vi "Main VI.vi"() -> ()   [LabVIEW 2017]
uses:
  State Machine Controler.ctl
  <vilib>/DAQmx/read.llb/DAQmx Read (Analog 1D DBL 1Chan NSamp).vi
  <vilib>/DAQmx/write.llb/DAQmx Write (Digital 1D Bool NChan 1Samp 1Line).vi
  <vilib>/DAQmx/miscellaneous.llb/DAQmx Fill In Error Info.vi
  <vilib>/DAQmx/create/channels.llb/DAQmx Create Channel (DO-Digital Output).vi
  <vilib>/DAQmx/configure/timing.llb/DAQmx Timing (Sample Clock).vi
panel:
  in  "BSL Flash 2":bool
  out "Auto Command indicator 3":u32
  out "Waveform Graph":dbl[](graph)
  out "output cluster":cluster{"x/y 2":dbl}(graph)
  out "Current loop count":i32
  out "Current value":dbl
  in  "physical channels":tag
  in  "error in":errorcluster
  out "Auto Command indicator 2":u32
  in  "BSL Flash wait time":u32=75
  out "Manual down  ON time":u32
  out "Auto Command indicator":u32
  out "Numeric":i32
  out "Auot Travel Time Indicator":u32
  in  "Auto Travel Time Controler":u32
  in  "Manual Up":bool
  in  "Manual Down":bool
  in  "Clamp/ Unclamp":bool
  out "State":T1
  in  "Auto Down Command":u32=75
  in  "Manual UP":bool
  in  "Stop":bool
  in  "BSL Flash":bool
  in  "Auto Down":bool
  in  "Auto UP":bool
  in  "Manual DOWN":bool
  # "Std Motor"
  # "Anti-Pinch Motor"
  # "min 87"
  # "max=526"
  # "max 537"
  # "Min=75"
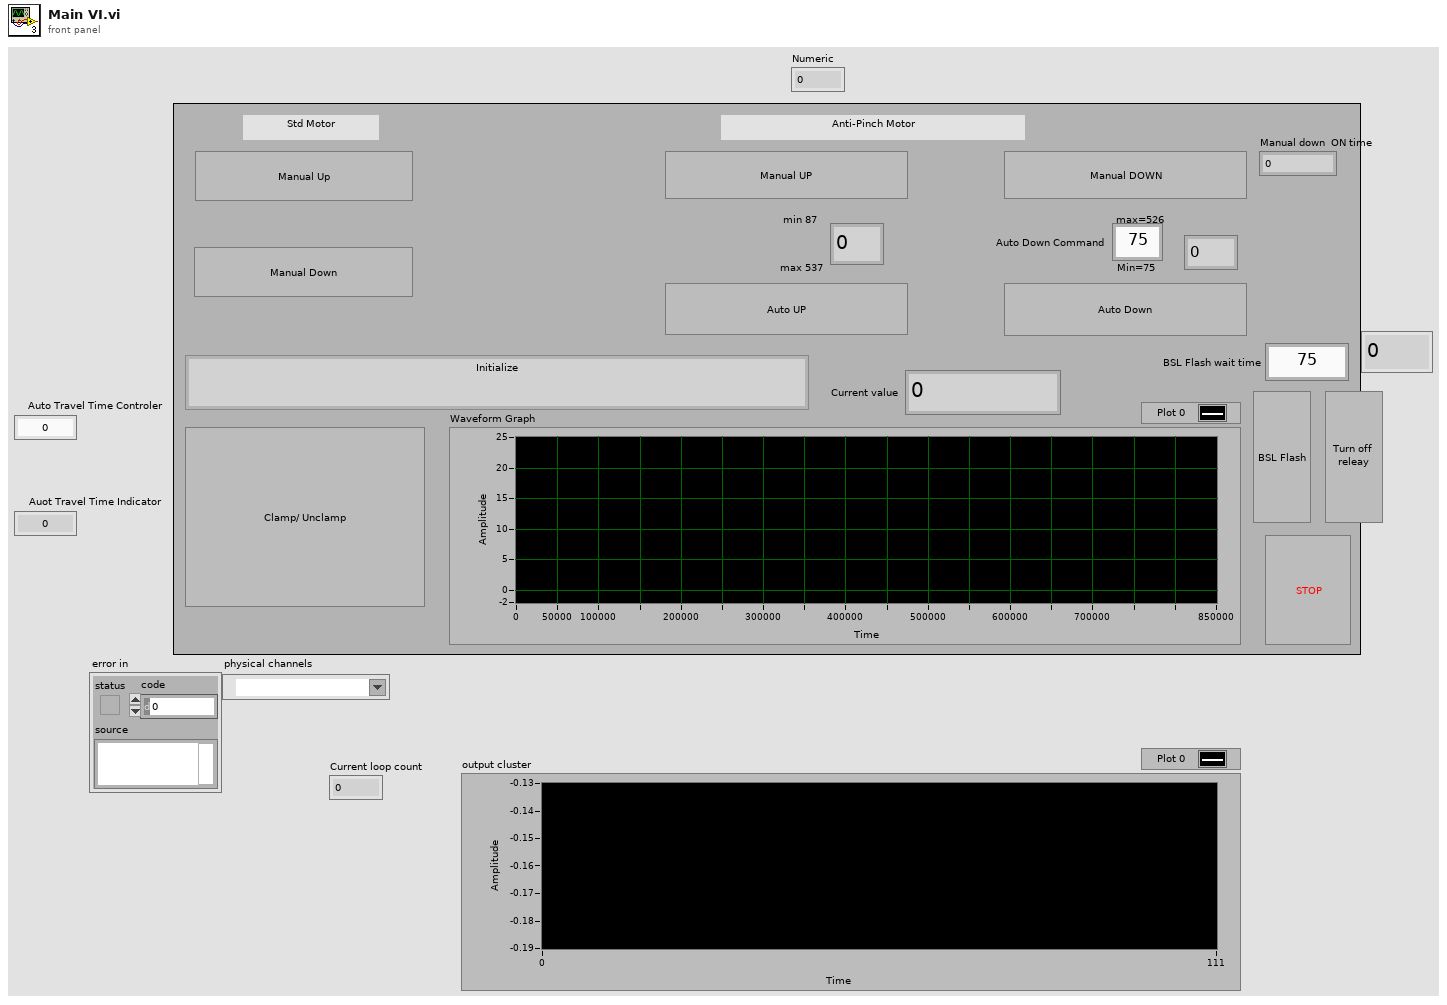
[diagram p1: front panel]
types:
  T1 = typedef "State Machine Controler.ctl" = enum16{"Initialize", "Wait for Action", "Manual Up AP", "Manual Up Std", "Manual Stop", "Manual Down AP", "Manual Down Std", "Auto Up", "Auto Down", "Auto Mode Down", "Auto Mode Up", "Auto Mode Waiting", "BSL Flash", "Stop"}
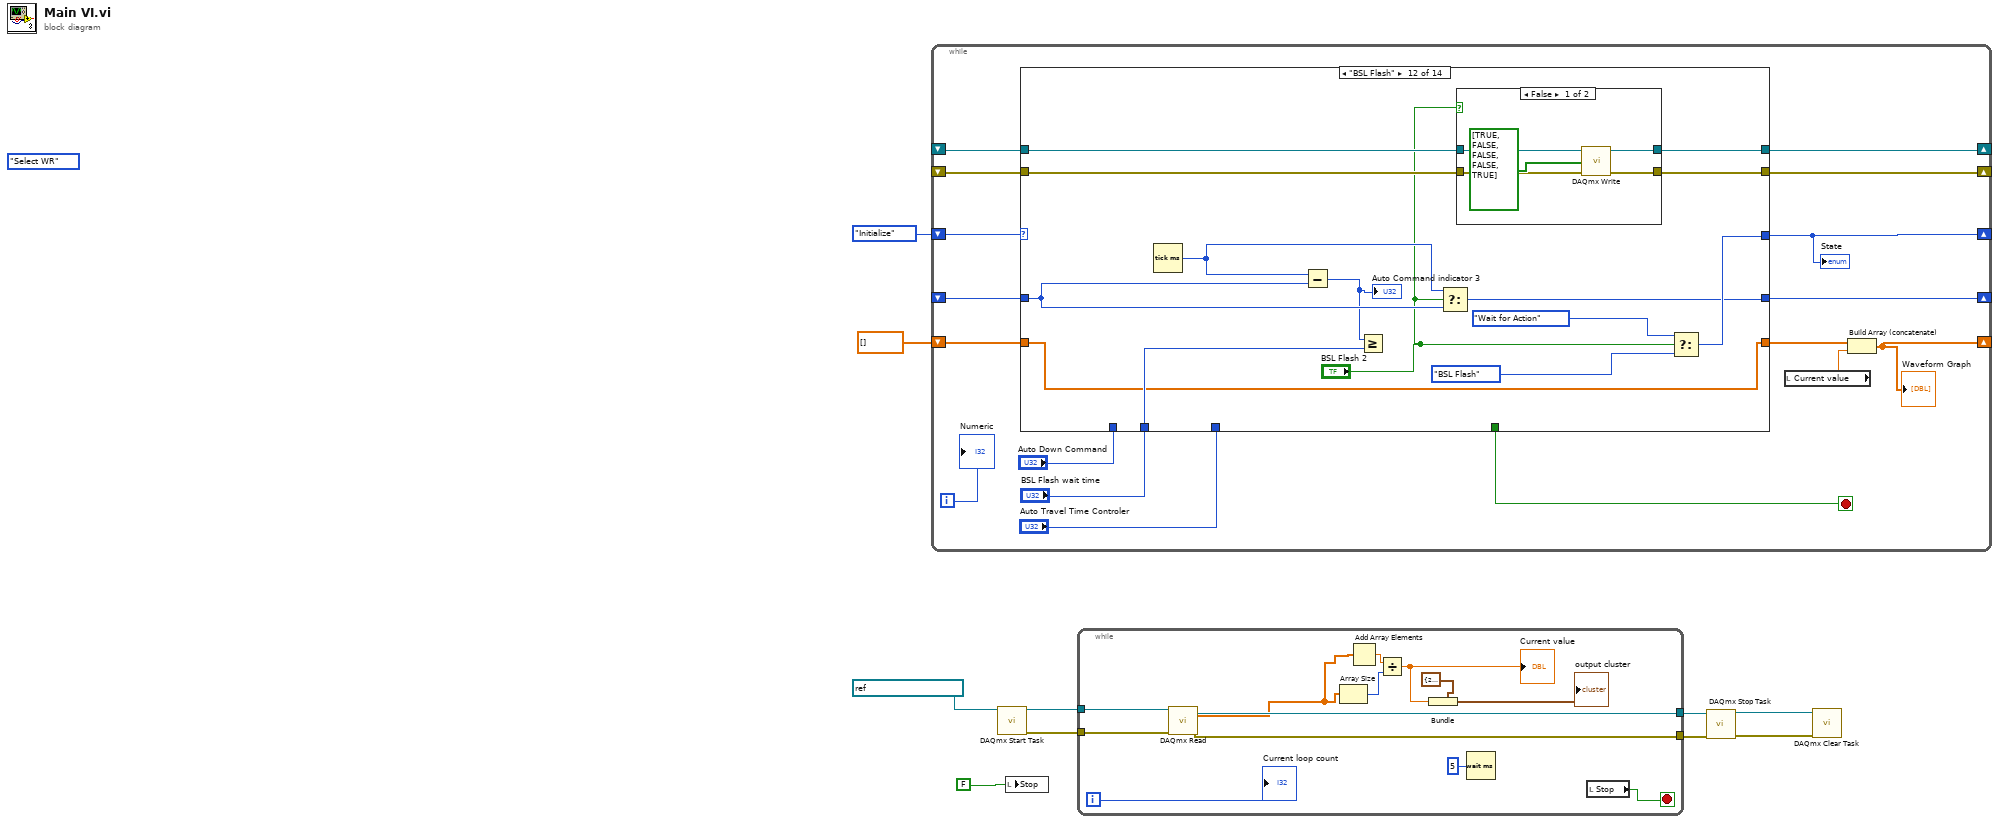
[diagram p0: block diagram]
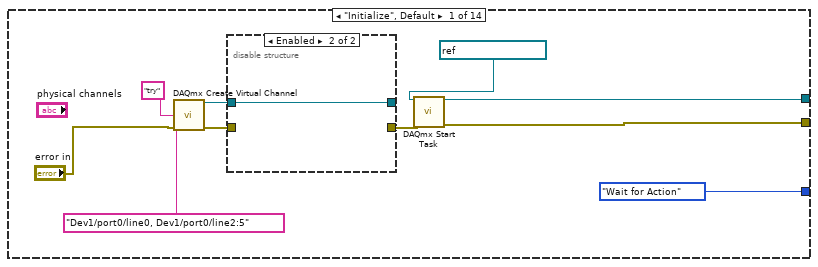
[diagram p2: hidden frame]
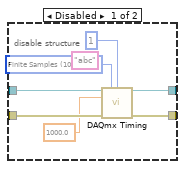
[diagram p3: hidden frame]
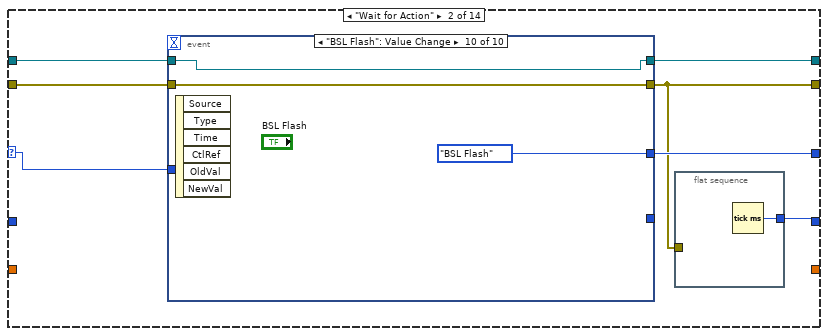
[diagram p4: hidden frame]
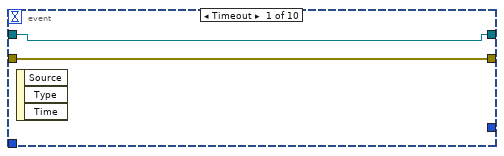
[diagram p5: hidden frame]
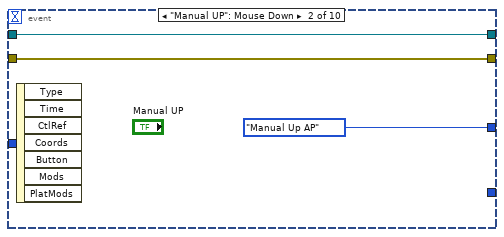
[diagram p6: hidden frame]
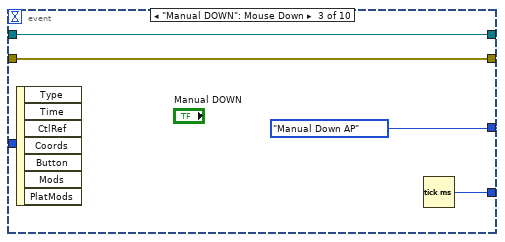
[diagram p7: hidden frame]
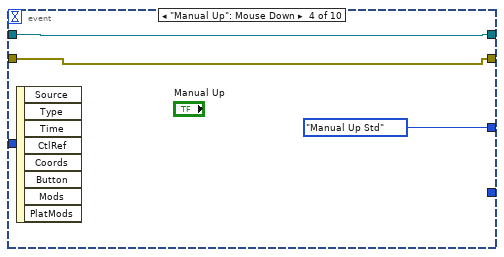
[diagram p8: hidden frame]
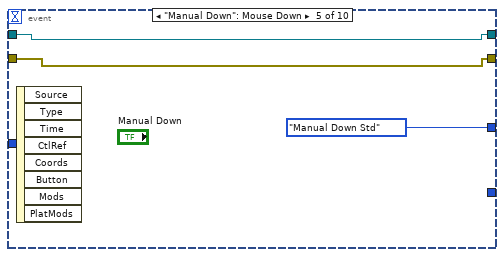
[diagram p9: hidden frame]
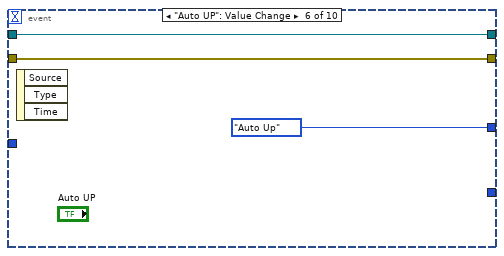
[diagram p10: hidden frame]
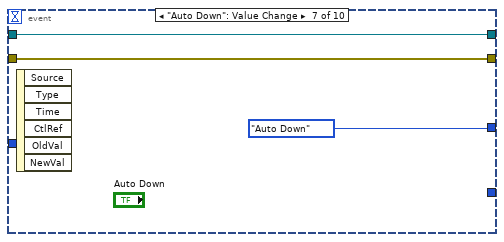
[diagram p11: hidden frame]
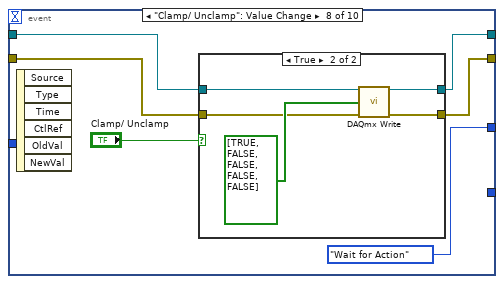
[diagram p12: hidden frame]
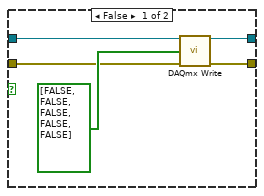
[diagram p13: hidden frame]
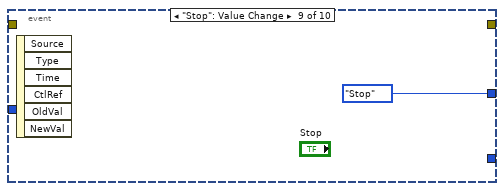
[diagram p14: hidden frame]
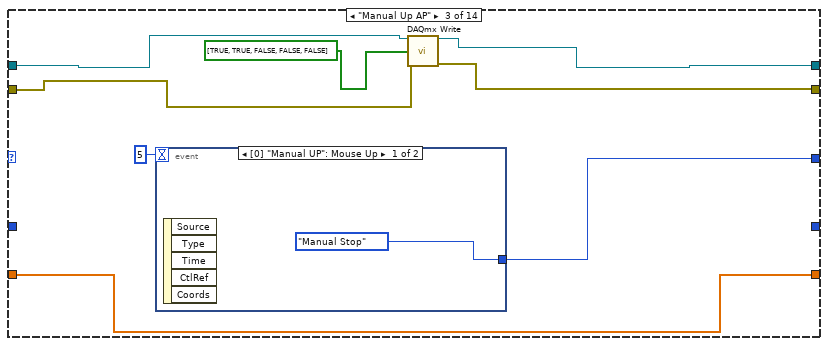
[diagram p15: hidden frame]
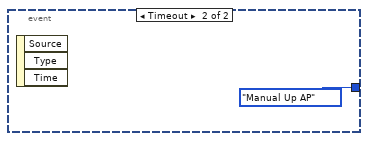
[diagram p16: hidden frame]
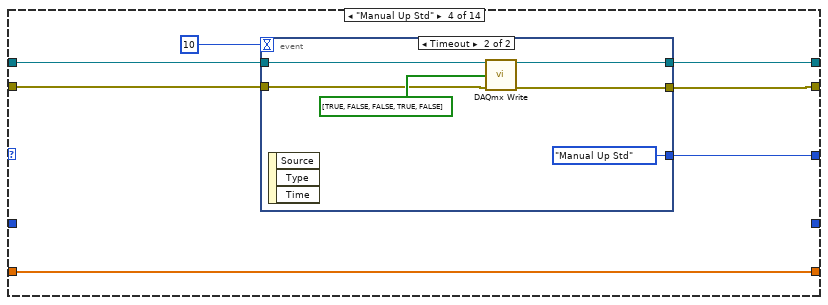
[diagram p17: hidden frame]
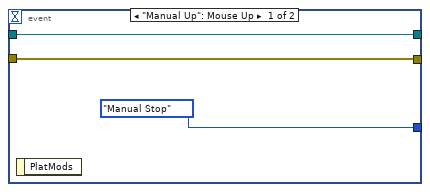
[diagram p18: hidden frame]
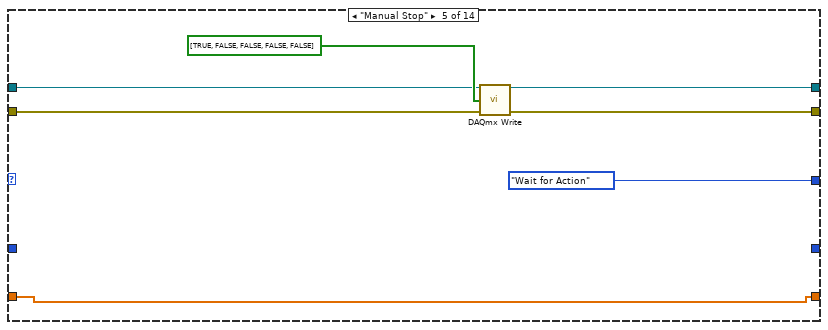
[diagram p19: hidden frame]
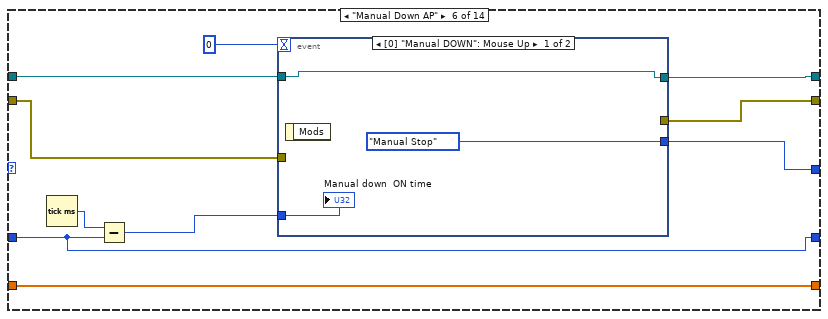
[diagram p20: hidden frame]
diagram:
  (unwired) enum16{"Select WR"}."Select WR"
  n1 = while {
    shift-right: [w18] -> _
    shift-left: State_Machine_Controler."Initialize" -> [w27]
    shift-right: [w22] -> _
    shift-left: _ -> [w24]
    shift-right: [w21] -> _
    shift-left: _ -> [w23]
    shift-right: [w26] -> _
    shift-left: _ -> [w25]
    shift-right: [w11] -> _
    shift-left: dbl[] [] -> [w14]
    i -> [w16]
    stop <- w20 stop-if-true
    n2 = case shown="\"BSL Flash\"" w27 {
      selector: w27 -> [_ w49 _ _ _ _ _ _ _ _ _ _ _ _]
      tunnel: [State_Machine_Controler."Wait for Action" w52 w102 w111 State_Machine_Controler."Wait for Action" w137 w153 State_Machine_Controler."Auto Mode Up" State_Machine_Controler."Auto Mode Down" w191 w212 w233 w252 State_Machine_Controler."Stop"] -> w18
      tunnel: w24 -> [_ w51 w100 w110 w126 w136 w152 w168 w178 w188 w210 w231 w258 w275]
      tunnel: w23 -> [_ w50 w99 w108 w125 w134 w150 w165 w177 w187 w209 w230 w257 w274]
      tunnel: [_ w46 _ _ _ w129 _ w170 w173 w182 w204 w226 w245 _] -> w26
      tunnel: w25 -> [_ _ _ _ _ w129 _ _ _ w181 w203 w225 w245 _]
      tunnel: "Auto Down Command" -> [_ _ _ _ _ _ _ _ _ w190 _ _ _ _]
      tunnel: [w36 w48 w97 w109 w123 w135 w151 w167 w175 w186 w208 w229 w255 _] -> w22
      tunnel: [w37 w47 w98 w107 w124 w133 w149 w164 w176 w185 w207 w228 w256 w271] -> w21
      tunnel: [_ _ _ _ _ _ _ _ _ _ _ _ _ TRUE ("Stop")] -> w20
      tunnel: "Auto Travel Time Controler" -> [_ _ _ _ _ _ _ _ _ _ _ _ w259 _]
      tunnel: "BSL Flash wait time" -> [_ _ _ _ _ _ _ _ _ _ w202 w224 _ _]
      tunnel: w14 -> [_ _ w96 w105 w121 w128 w147 w163 w171 w179 w200 w222 w251 _]
      tunnel: [_ _ w96 w105 w121 w128 w147 w163 w171 w179 w200 w222 w251 _] -> w12
      frame "Initialize", Default {
        n3 = call-poly <vilib>:"DAQmx Create Virtual Channel.vi"("lines"=tag "Dev1/port0/line0, Dev1/port0/line2:5", "name to assign"="try", "error in"="error in") -> ("task out"=w31:refnum<k21>, "error out"=w30:errorcluster)  [unwired: 11 in]
        n4 = disable-structure shown="Enabled" {
          disable-tunnel: w31 -> [w44 w45]
          disable-tunnel: [w43 w45] -> _
          disable-tunnel: w30 -> [w41 _]
          disable-tunnel: [w40 _] -> w29
          frame Disabled {
            w42 = 10178 items=["Finite Samples"=10178, "Continuous Samples"=10123, "Hardware Timed Single Point"=12522] ("sample mode")
            (unwired) "abc" ("new task name")
            n5 = call-poly <vilib>:"DAQmx Timing.vi"("task/channels in"=w44, "sample mode"=w42, "samples per channel"=1, "rate"=1000.0, "error in"=w41) -> ("task out"=w43:refnum<k21>, "error out"=w40:errorcluster)  [unwired: 9 in]
          }
          frame Enabled {
          }
        }
        n6 = call <vilib>:"DAQmx Start Task.vi"("task/channels in"=refnum<k21> "Test AP UP_DN", "error in"=w29) -> ("task out"=w36:refnum<k21>, "error out"=w37:errorcluster)  [unwired: 12 in]
      }
      frame "Wait for Action" {
        n7 = event shown="[9] \"BSL Flash\": Value Change" {
          selector: _ -> [_ _ _ _ _ _ _ _ _ _]
          dyn-events: _ -> [_ _ _ _ _ _ _ _ _ _]
          timeout: _ -> [_ _ _ _ _ _ _ _ _ _]
          tunnel: [_ State_Machine_Controler."Manual Up AP" State_Machine_Controler."Manual Down AP" State_Machine_Controler."Manual Up Std" State_Machine_Controler."Manual Down Std" State_Machine_Controler."Auto Up" State_Machine_Controler."Auto Down" State_Machine_Controler."Wait for Action" State_Machine_Controler."Stop" State_Machine_Controler."BSL Flash"] -> w52
          tunnel: w51 -> [w55 w57 w61 w64 w67 w69 w74 w80 _ w93]
          tunnel: w50 -> [w54 w56 w60 w63 w66 w70 w73 w78 _ w92]
          tunnel: [w55 w57 w61 w64 w67 w69 w74 w79 _ w93] -> w48
          tunnel: [w54 w56 w60 w63 w66 w70 w73 w77 _ w92] -> w47
          tunnel: w49 -> [_ _ _ _ _ _ _ _ _ _]
          tunnel: [_ _ w59 _ _ _ _ _ _ _] -> _
          event Timeout {
            n8 = event-data() -> ()  [unwired: 1 in, 3 out]
          }
          event "Manual UP": Mouse Down {
            n9 = event-data() -> ()  [unwired: 1 in, 7 out]
          }
          event "Manual DOWN": Mouse Down {
            n10 = event-data() -> ()  [unwired: 1 in, 7 out]
            n11 = Tick Count (ms)() -> (millisecond timer value=w59:u32)
          }
          event "Manual Up": Mouse Down {
            n12 = event-data() -> ()  [unwired: 1 in, 8 out]
          }
          event "Manual Down": Mouse Down {
            n13 = event-data() -> ()  [unwired: 1 in, 8 out]
          }
          event "Auto UP": Value Change {
            n14 = event-data() -> ()  [unwired: 1 in, 3 out]
          }
          event "Auto Down": Value Change {
            n15 = event-data() -> ()  [unwired: 1 in, 6 out]
          }
          event "Clamp/ Unclamp": Value Change {
            n16 = event-data() -> ()  [unwired: 1 in, 6 out]
            n17 = case shown="True" "Clamp/ Unclamp" {
              tunnel: w80 -> [w84 w89]
              tunnel: [w83 w88] -> w79
              tunnel: w78 -> [w82 w87]
              tunnel: [w81 w86] -> w77
              frame False {
                n18 = call-poly <vilib>:"DAQmx Write.vi"("task/channels in"=w84, "data"=bool[] [FALSE, FALSE, FALSE, FALSE, FALSE], "error in"=w82) -> ("task out"=w83:refnum<k21>, "error out"=w81:errorcluster)  [unwired: 10 in, 1 out]
              }
              frame True {
                n19 = call-poly <vilib>:"DAQmx Write.vi"("task/channels in"=w89, "data"=bool[] [TRUE, FALSE, FALSE, FALSE, FALSE], "error in"=w87) -> ("task out"=w88:refnum<k21>, "error out"=w86:errorcluster)  [unwired: 10 in, 1 out]
              }
            }
          }
          event "Stop": Value Change {
            n20 = event-data() -> ()  [unwired: 1 in, 6 out]
          }
          event "BSL Flash": Value Change {
            n21 = event-data() -> ()  [unwired: 1 in, 6 out]
          }
        }
        n22 = flat-sequence {
          tunnel: w47 -> [_]
          tunnel: [w53] -> w46
          frame #0 {
            n23 = Tick Count (ms)() -> (millisecond timer value=w53:u32)
          }
        }
      }
      frame "Manual Up AP" {
        n24 = event shown="[0] \"Manual UP\": Mouse Up" {
          selector: _ -> [_ _]
          dyn-events: _ -> [_ _]
          timeout: 5 -> [_ _]
          tunnel: [State_Machine_Controler."Manual Stop" State_Machine_Controler."Manual Up AP"] -> w102
          event "Manual UP": Mouse Up {
            n25 = event-data() -> ()  [unwired: 1 in, 5 out]
          }
          event Timeout {
            n26 = event-data() -> ()  [unwired: 1 in, 3 out]
          }
        }
        n27 = call-poly <vilib>:"DAQmx Write.vi"("task/channels in"=w100, "data"=bool[] [TRUE, TRUE, FALSE, FALSE, FALSE], "error in"=w99) -> ("task out"=w97:refnum<k21>, "error out"=w98:errorcluster)  [unwired: 10 in, 1 out]
      }
      frame "Manual Up Std" {
        n28 = event shown="[1] Timeout" {
          selector: _ -> [_ _]
          dyn-events: _ -> [_ _]
          timeout: 10 -> [_ _]
          tunnel: [State_Machine_Controler."Manual Stop" State_Machine_Controler."Manual Up Std"] -> w111
          tunnel: w110 -> [w113 w119]
          tunnel: [w113 w118] -> w109
          tunnel: w108 -> [w112 w117]
          tunnel: [w112 w116] -> w107
          event "Manual Up": Mouse Up {
            n29 = event-data() -> ()  [unwired: 1 in, 1 out]
          }
          event Timeout {
            n30 = event-data() -> ()  [unwired: 1 in, 3 out]
            n31 = call-poly <vilib>:"DAQmx Write.vi"("task/channels in"=w119, "data"=bool[] [TRUE, FALSE, FALSE, TRUE, FALSE], "error in"=w117) -> ("task out"=w118:refnum<k21>, "error out"=w116:errorcluster)  [unwired: 10 in, 1 out]
          }
        }
      }
      frame "Manual Stop" {
        n32 = call-poly <vilib>:"DAQmx Write.vi"("task/channels in"=w126, "data"=bool[] [TRUE, FALSE, FALSE, FALSE, FALSE], "error in"=w125) -> ("task out"=w123:refnum<k21>, "error out"=w124:errorcluster)  [unwired: 10 in, 1 out]
      }
      frame "Manual Down AP" {
        n33 = Tick Count (ms)() -> (millisecond timer value=w131:u32)
        n34 = Subtract(x=w131, y=w129) -> (x-y=w130:u32)
        n35 = event shown="[0] \"Manual DOWN\": Mouse Up" {
          selector: _ -> [_ _]
          dyn-events: _ -> [_ _]
          timeout: 0 -> [_ _]
          tunnel: [State_Machine_Controler."Manual Stop" State_Machine_Controler."Manual Down AP"] -> w137
          tunnel: w136 -> [w139 w145]
          tunnel: [w139 w144] -> w135
          tunnel: w134 -> [_ w143]
          tunnel: [_ w142] -> w133
          tunnel: w130 -> [w138 _]
          event "Manual DOWN": Mouse Up {
            n36 = event-data() -> ()  [unwired: 1 in, 1 out]
            "Manual down  ON time" <- w138
          }
          event Timeout {
            n37 = event-data() -> ()  [unwired: 1 in, 3 out]
            n38 = call-poly <vilib>:"DAQmx Write.vi"("task/channels in"=w145, "data"=bool[] [TRUE, FALSE, TRUE, FALSE, FALSE], "error in"=w143) -> ("task out"=w144:refnum<k21>, "error out"=w142:errorcluster)  [unwired: 10 in, 1 out]
          }
        }
      }
      frame "Manual Down Std" {
        n39 = event shown="[1] Timeout" {
          selector: _ -> [_ _]
          dyn-events: _ -> [_ _]
          timeout: 10 -> [_ _]
          tunnel: [State_Machine_Controler."Manual Stop" State_Machine_Controler."Manual Down Std"] -> w153
          tunnel: w152 -> [w155 w160]
          tunnel: [w155 w159] -> w151
          tunnel: w150 -> [w154 w158]
          tunnel: [w154 w157] -> w149
          event "Manual Down": Mouse Up {
            n40 = event-data() -> ()  [unwired: 1 in, 5 out]
          }
          event Timeout {
            n41 = event-data() -> ()  [unwired: 1 in, 3 out]
            n42 = call-poly <vilib>:"DAQmx Write.vi"("task/channels in"=w160, "data"=bool[] [TRUE, FALSE, FALSE, FALSE, TRUE], "error in"=w158) -> ("task out"=w159:refnum<k21>, "error out"=w157:errorcluster)  [unwired: 10 in, 1 out]
          }
        }
      }
      frame "Auto Up" {
        n43 = call-poly <vilib>:"DAQmx Write.vi"("task/channels in"=w168, "data"=bool[] [TRUE, TRUE, FALSE, FALSE, FALSE], "error in"=w165) -> ("task out"=w167:refnum<k21>, "error out"=w164:errorcluster)  [unwired: 10 in, 1 out]
        n44 = Tick Count (ms)() -> (millisecond timer value=w170:u32)
      }
      frame "Auto Down" {
        n45 = call-poly <vilib>:"DAQmx Write.vi"("task/channels in"=w178, "data"=bool[] [TRUE, FALSE, TRUE, FALSE, FALSE], "error in"=w177) -> ("task out"=w175:refnum<k21>, "error out"=w176:errorcluster)  [unwired: 10 in, 1 out]
        n46 = Tick Count (ms)() -> (millisecond timer value=w173:u32)
      }
      frame "Auto Mode Down" {
        n47 = Tick Count (ms)() -> (millisecond timer value=w183:u32)
        n48 = Subtract(x=w183, y=w181) -> (x-y=w180:u32)
        "Auto Command indicator 2" <- w180
        n49 = Greater Or Equal?(x=w180, y=w190) -> (x >= y?=w184:bool)
        n50 = Select(t=w183, s=w184, f=w181) -> (s? t:f=w182:u32)
        n51 = case shown="True" w184 {
          tunnel: w188 -> [w196 w199]
          tunnel: w187 -> [w195 w198]
          tunnel: [w194 w199] -> w186
          tunnel: [w193 w198] -> w185
          frame True {
            n52 = call-poly <vilib>:"DAQmx Write.vi"("task/channels in"=w196, "data"=bool[] [TRUE, FALSE, FALSE, FALSE, FALSE], "error in"=w195) -> ("task out"=w194:refnum<k21>, "error out"=w193:errorcluster)  [unwired: 10 in, 1 out]
          }
          frame False {
          }
        }
        n53 = Select(t=State_Machine_Controler."Auto Mode Waiting", s=w184, f=State_Machine_Controler."Auto Mode Down") -> (s? t:f=w191:T1)
      }
      frame "Auto Mode Up" {
        n54 = Tick Count (ms)() -> (millisecond timer value=w205:u32)
        n55 = Subtract(x=w205, y=w203) -> (x-y=w201:u32)
        "Auto Command indicator" <- w201
        n56 = Greater Or Equal?(x=w201, y=w202) -> (x >= y?=w206:bool)
        n57 = Select(t=w205, s=w206, f=w203) -> (s? t:f=w204:u32)
        n58 = case shown="True" w206 {
          tunnel: w210 -> [w217 w220]
          tunnel: w209 -> [w216 w219]
          tunnel: [w215 w220] -> w208
          tunnel: [w214 w219] -> w207
          frame True {
            n59 = call-poly <vilib>:"DAQmx Write.vi"("task/channels in"=w217, "data"=bool[] [TRUE, FALSE, FALSE, FALSE, FALSE], "error in"=w216) -> ("task out"=w215:refnum<k21>, "error out"=w214:errorcluster)  [unwired: 10 in, 1 out]
          }
          frame False {
          }
        }
        n60 = Select(t=State_Machine_Controler."Auto Mode Waiting", s=w206, f=State_Machine_Controler."Auto Mode Up") -> (s? t:f=w212:T1)
      }
      frame "BSL Flash" {
        n61 = Tick Count (ms)() -> (millisecond timer value=w227:u32)
        n62 = Subtract(x=w227, y=w225) -> (x-y=w223:u32)
        "Auto Command indicator 3" <- w223
        n63 = Greater Or Equal?(x=w223, y=w224) -> ()  [unwired: 1 out]
        n64 = Select(t=w227, s="BSL Flash 2", f=w225) -> (s? t:f=w226:u32)
        n65 = case shown="False" "BSL Flash 2" {
          tunnel: w231 -> [w238 w243]
          tunnel: w230 -> [w237 w242]
          tunnel: [w236 w241] -> w229
          tunnel: [w235 w240] -> w228
          frame False {
            n66 = call-poly <vilib>:"DAQmx Write.vi"("task/channels in"=w238, "data"=bool[] [TRUE, FALSE, FALSE, FALSE, TRUE], "error in"=w237) -> ("task out"=w236:refnum<k21>, "error out"=w235:errorcluster)  [unwired: 10 in, 1 out]
          }
          frame True {
            n67 = call-poly <vilib>:"DAQmx Write.vi"("task/channels in"=w243, "data"=bool[] [TRUE, FALSE, FALSE, FALSE, FALSE], "error in"=w242) -> ("task out"=w241:refnum<k21>, "error out"=w240:errorcluster)  [unwired: 10 in, 1 out]
          }
        }
        n68 = Select(t=State_Machine_Controler."Wait for Action", s="BSL Flash 2", f=State_Machine_Controler."BSL Flash") -> (s? t:f=w233:T1)
      }
      frame "Auto Mode Waiting" {
        n69 = Tick Count (ms)() -> (millisecond timer value=w261:u32)
        n70 = Subtract(x=w261, y=w245) -> (x-y=w260:u32)
        "Auot Travel Time Indicator" <- w260
        n71 = Greater Or Equal?(x=w260, y=w259) -> (x >= y?=w247:bool)
        n72 = local read "Current value"() -> (w250:dbl)
        n73 = case shown="True" w247 {
          tunnel: w258 -> [w263 w268]
          tunnel: w257 -> [w262 w267]
          tunnel: [w262 w266] -> w256
          tunnel: [w263 w265] -> w255
          frame False {
          }
          frame True {
            n74 = call-poly <vilib>:"DAQmx Write.vi"("task/channels in"=w268, "data"=bool[] [TRUE, FALSE, FALSE, FALSE, FALSE], "error in"=w267) -> ("task out"=w265:refnum<k21>, "error out"=w266:errorcluster)  [unwired: 10 in, 1 out]
          }
        }
        n75 = Less?(x=w250, y=1.0) -> (x < y?=w248:bool)
        n76 = Compound Arithmetic op=AND(w248, w247) -> (w246:bool)
        n77 = Select(t=State_Machine_Controler."Wait for Action", s=w246, f=State_Machine_Controler."Auto Mode Waiting") -> (s? t:f=w252:T1)
      }
      frame "Stop" {
        n78 = call <vilib>:"DAQmx Stop Task.vi"("task/channels in"=w275, "error in"=w274) -> ("task out"=w272:refnum<k21>, "error out"=w273:errorcluster)  [unwired: 12 in]
        n79 = call <vilib>:"DAQmx Clear Task.vi"("task in"=w272, "error in"=w273) -> ("error out"=w271:errorcluster)  [unwired: 13 in]
      }
    }
    "State" <- w18
    n80 = local read "Current value"() -> (w13:dbl)
    n81 = Build Array (concatenate)(w12, w13) -> (w11:dbl[])
    "Waveform Graph" <- w11
    "Numeric" <- w16
  }
  n82 = call <vilib>:"DAQmx Start Task.vi"("task/channels in"=refnum<k21> "1922_601_Current") -> ("task out"=w8:refnum<k21>, "error out"=w7:errorcluster)  [unwired: 13 in]
  n83 = local write "Stop"(FALSE) -> ()
  n84 = while {
    tunnel: w8 -> [w288]
    tunnel: w7 -> [w287]
    tunnel: [w286] -> w6
    tunnel: [w285] -> w5
    i -> [w280]
    stop <- w281 stop-if-true
    n85 = call-poly <vilib>:"DAQmx Read.vi"("task/channels in"=w288, "error in"=w287) -> ("task out"=w286:refnum<k21>, "data"=w283:dbl[], "error out"=w285:errorcluster)  [unwired: 11 in]
    n86 = Array Size(array=w283) -> (size(s)=w284:i32)
    n87 = Add Array Elements(numeric array=w283) -> (sum=w282:dbl)
    n88 = Divide(x=w282, y=w284) -> (x/y=w277:dbl)
    "Current value" <- w277
    n89 = Bundle(cluster=cluster{"x/y 2":dbl} {"x/y 2"=2.5136913175241347}, "x/y 2"=w277) -> (→"output cluster":cluster{"x/y 2":dbl})
    n90 = Wait (ms)(milliseconds to wait=u32 5) -> ()  [unwired: 1 out]
    n91 = local read "Stop"() -> (w281:bool)
    "Current loop count" <- w280
  }
  n92 = call <vilib>:"DAQmx Stop Task.vi"("task/channels in"=w6, "error in"=w5) -> ("task out"=w4:refnum<k21>, "error out"=w3:errorcluster)  [unwired: 12 in]
  n93 = call <vilib>:"DAQmx Clear Task.vi"("task in"=w4, "error in"=w3) -> ()  [unwired: 13 in, 1 out]
